vi "[GV]_IMU yaw.vi"() -> ()   [LabVIEW 2016]
panel:
  out "IMU_Yaw":dbl
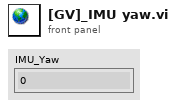
[diagram p1: front panel]
diagram:
